vi "Add NI-XNET CAN Hardware_Add Log File_Add Trigger.vi"(7 "SysDef Ref":T1, 8 "error in (no error)":errorcluster, 10 "Trigger Node Path":string, 11 "Log File Ref":refnum<k24>) -> (0 "error out":errorcluster, 3 "Log File Ref out":refnum<k24>)   [LabVIEW 2019, in "Simple SysDef API.lvlib"]
uses:
  <userlib>/SimpleSysDef/Simple SysDef API.lvlib
  NationalInstruments.VeriStand.SystemDefinitionAPI
  <userlib>/SimpleSysDef/_SubVIs/System Definition Reference.ctl
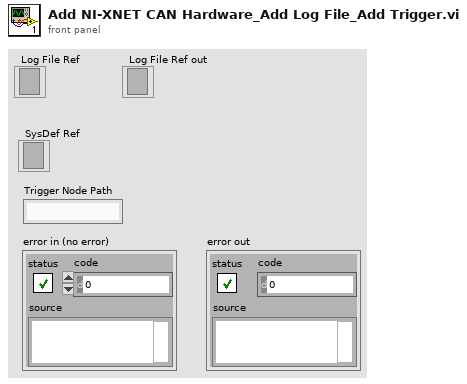
[diagram p1: front panel]
types:
  T1 = typedef "Simple SysDef API.lvlib/System Definition Reference.ctl" = refnum<k24>
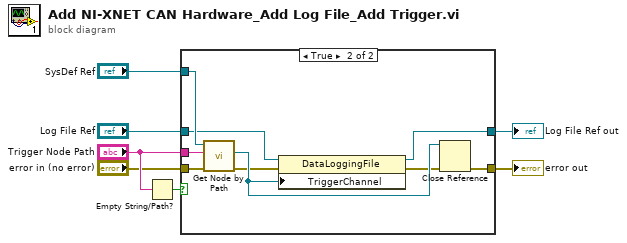
[diagram p0: block diagram]
diagram:
  n1 = Empty String/Path?(string/path="Trigger Node Path") -> (empty?=w5:bool)
  n2 = case shown="True" w5 {
    tunnel: [w9 w15] -> w6
    tunnel: "Log File Ref" -> [w8 w14]
    tunnel: "error in (no error)" -> [w9 w18]
    tunnel: "Trigger Node Path" -> [_ w17]
    tunnel: "SysDef Ref" -> [_ w16]
    tunnel: [w8 w10] -> w1
    frame False {
    }
    frame True {
      n3 = call <userlib>:"Get Node by Path.vi"("error in (no error)"=w18, "System Definition Node Path"=w17, "SysDef Ref"=w16) -> ("error out"=w12:errorcluster, "Node Ref"=w13:refnum<k24>)  [unwired: 6 in, 1 out]
      n4 = property class="DataLoggingFile"(reference=w14, error in=w12, "TriggerChannel"=w13) -> (reference out=w10:refnum<k24>, error out=w11:errorcluster)
      n5 = Close Reference(reference=w13, error in (no error)=w11) -> (error out=w15:errorcluster)
    }
  }
  "Log File Ref out" <- w1
  "error out" <- w6
